vi "Configure RemIO Module Core.vi"(8 "error in (no error)":errorcluster, 9 "module slot index":u8=1, 10 "Slave Ref In":refnum<k21>, 11 "11154 in":refnum<class "11154.lvclass">) -> (0 "error out":errorcluster, 1 "negative confirmation":T1 {"additional error code" format="%.0x"; "error code" format="%.0x"}, 2 "Slave Ref Out":refnum<k21>, 3 "11154 out":refnum<class "11154.lvclass">, 5 "SDO abort code":u32 format="%.0x")   [LabVIEW 2017, in "Modules.lvlib" / "11154.lvclass"]
uses:
  11154.lvclass
  <vilib>/indcomecat/Remote IO/typedefs/negative confirmation.ctl
  11154.lvclass/11154.ctl
  <vilib>/indcomecat/Remote IO/internal/_Configure REM-11154.vi
  <vilib>/indcomecat/Remote IO/NI ECAT Remote IO.lvlib
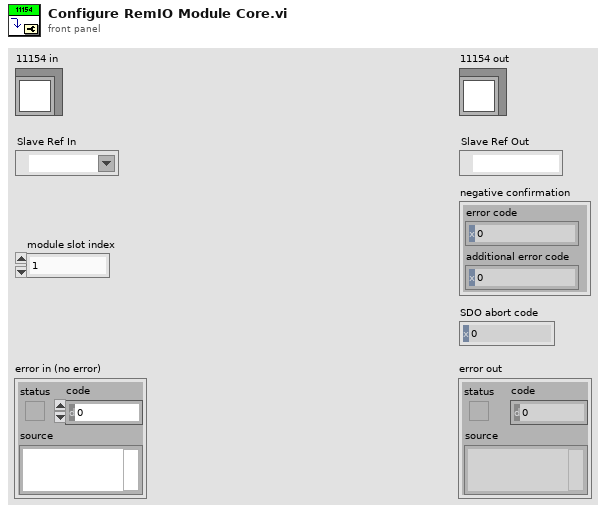
[diagram p1: front panel]
types:
  T1 = typedef "negative confirmation.ctl" = cluster{"error code":u16, "additional error code":u16}
  T2 = typedef "NI ECAT Remote IO.lvlib/input filter time REM-11154.ctl" = u8
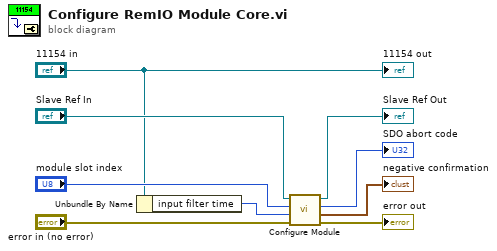
[diagram p0: block diagram]
diagram:
  n1 = Unbundle By Name("11154 in") -> ("input filter time"=w1:T2)
  n2 = call-poly <vilib>:"Configure Module.vi"("error in (no error)"="error in (no error)", "input filter time"=w1, "module slot index"="module slot index", "slave reference in"="Slave Ref In") -> ("error out"=→"error out":errorcluster, "negative confirmation"=→"negative confirmation":T1, "SDO abort code"=→"SDO abort code":u32, "slave reference out"=→"Slave Ref Out":refnum<k21>)  [unwired: 4 in]
  "11154 out" <- "11154 in"
